vi "Print Error.vi"(5 "Custom Device? (T)":bool=TRUE, 7 "error in (no error)":errorcluster, 9 "Note (empty)":string, 10 "Your code's public name":string) -> (0 "error out":errorcluster)   [LabVIEW 2019, in "Scan Engine Custom Device.lvlib"]
doc: "Prints error information out to the console. Provide your code's public name. For example, if your code is about J1939, put that here so the user knows what this printed error information has to do with.\n\nIf this is not a NI VeriStand custom device, write false to the Custom Device? input. This will change the error output and cause this to ignore error -2206.\n\nIf the 'note' field is empty, it is not printed to the console.\n\nExample output 1:\n******J1939 ERROR******\nSource: blah.vi\nCode: 535\n******J1939 ERROR******\n\nExample output 2:\n******XCP and CCP Master CUSTOM DEVICE ERROR******\nSource: blah.vi\nCode: 535\nUser Note: before write\n******XCP and CCP Master CUSTOM DEVICE ERROR******"
uses:
  Scan Engine Custom Device.lvlib
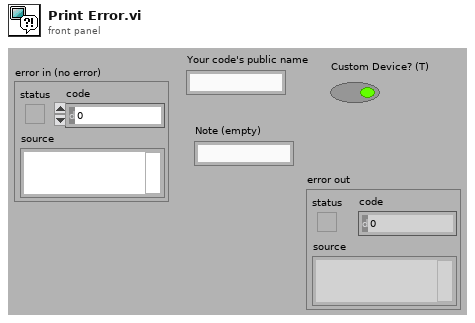
[diagram p1: front panel]
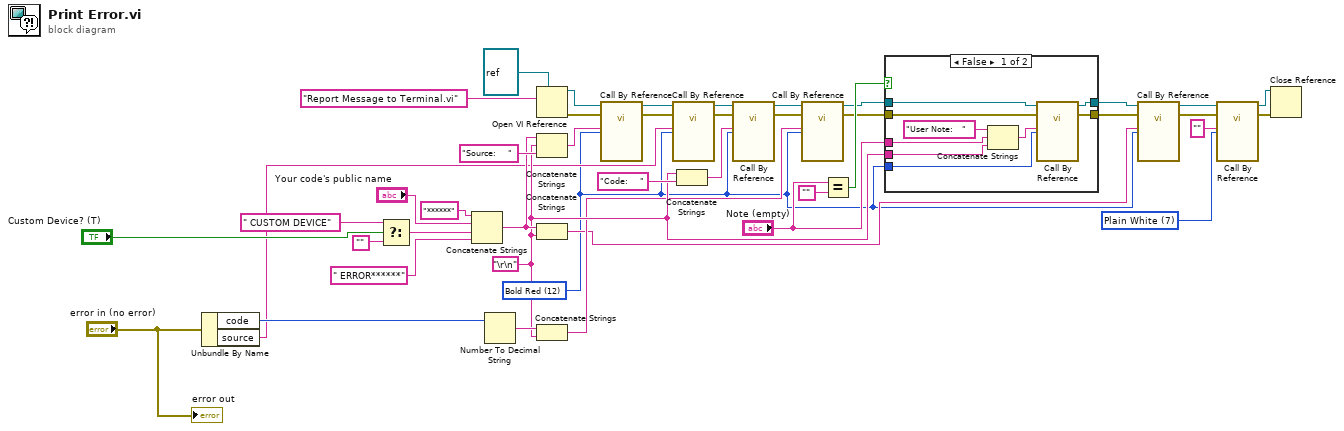
[diagram p0: block diagram]
diagram:
  w22 = u16 7 items=["Plain White"=7, "Bold White"=15, "Bold Blue"=9, "Bold Green"=10, "Bold Red"=12] ("Color (Plain White)")
  w2 = u16 12 items=["Plain White"=7, "Bold White"=15, "Bold Blue"=9, "Bold Green"=10, "Bold Red"=12] ("Color (Plain White)")
  w29 = "\r\n"
  n1 = Unbundle By Name("error in (no error)") -> ("code"=w41:i32, "source"=w19:string)
  n2 = Select(t=" CUSTOM DEVICE" ("String"), s="Custom Device? (T)", f="") -> (s? t:f=w27:string)
  n3 = Concatenate Strings("******" ("String"), "Your code's public name", w27, " ERROR******" ("String")) -> (w33:string)
  n4 = Number To Decimal String(number=w41) -> (decimal integer string=w38:string)  [unwired: 1 in]
  n5 = Open VI Reference(type specifier VI Refnum (for type only)=refnum<vi> refnum, vi path="Report Message to Terminal.vi") -> (vi reference=w17:refnum<vi>, error out=w16:errorcluster)  [unwired: 1 in, 3 out]
  n6 = Concatenate Strings(w33, w29, "Source:    " ("String")) -> (w21:string)
  n7 = Concatenate Strings(w33, w29) -> (w3:string)
  n8 = Concatenate Strings(w38, w29) -> (w12:string)
  n9 = call-by-ref "?"(reference=w17, error in=w16, "Color (Plain White)"=w2, "Message"=w21) -> (reference out=w18:refnum<vi>, error out=w20:errorcluster)  [unwired: 9 in, 1 out]
  n10 = call-by-ref "?"(reference=w18, error in=w20, "Color (Plain White)"=w2, "Message"=w19) -> (reference out=w13:refnum<vi>, error out=w14:errorcluster)  [unwired: 9 in, 1 out]
  n11 = Concatenate Strings(w29, "Code:    " ("String")) -> (w15:string)
  n12 = call-by-ref "?"(reference=w13, error in=w14, "Color (Plain White)"=w2, "Message"=w15) -> (reference out=w11:refnum<vi>, error out=w10:errorcluster)  [unwired: 9 in, 1 out]
  n13 = call-by-ref "?"(reference=w11, error in=w10, "Color (Plain White)"=w2, "Message"=w12) -> (reference out=w8:refnum<vi>, error out=w9:errorcluster)  [unwired: 9 in, 1 out]
  n14 = Equal?(x="Note (empty)", y="") -> (x = y?=w31:bool)
  n15 = case shown="False" w31 {
    tunnel: "Note (empty)" -> [w51 _]
    tunnel: w29 -> [w50 _]
    tunnel: [w47 w54] -> w7
    tunnel: w9 -> [w49 w54]
    tunnel: w8 -> [w46 w53]
    tunnel: [w45 w53] -> w4
    tunnel: w2 -> [w44 _]
    frame False {
      n16 = Concatenate Strings("User Note:   " ("string"), w51, w50) -> (w48:string)
      n17 = call-by-ref "?"(reference=w46, error in=w49, "Color (Plain White)"=w44, "Message"=w48) -> (reference out=w45:refnum<vi>, error out=w47:errorcluster)  [unwired: 9 in, 1 out]
    }
    frame True {
    }
  }
  n18 = call-by-ref "?"(reference=w4, error in=w7, "Color (Plain White)"=w2, "Message"=w3) -> (reference out=w5:refnum<vi>, error out=w6:errorcluster)  [unwired: 9 in, 1 out]
  n19 = call-by-ref "?"(reference=w5, error in=w6, "Color (Plain White)"=w22, "Message"="") -> (reference out=w23:refnum<vi>, error out=w24:errorcluster)  [unwired: 9 in, 1 out]
  n20 = Close Reference(reference=w23, error in (no error)=w24) -> ()  [unwired: 1 out]
  "error out" <- "error in (no error)"
